vi "limit switch.vi"(9 "lower limit":bool, 10 "upper limit":bool, 11 "motor input":dbl) -> (3 "motor output":dbl)   [LabVIEW 2014]
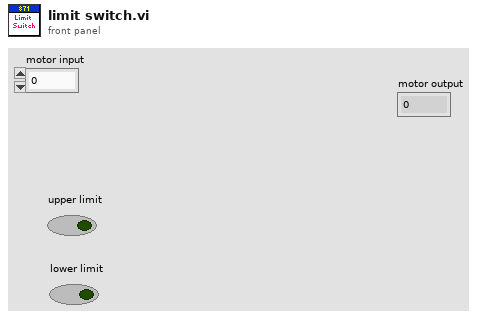
[diagram p1: front panel]
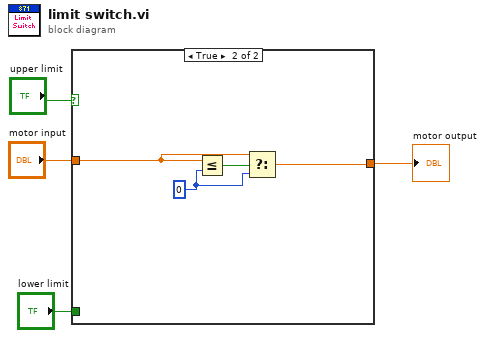
[diagram p0: block diagram]
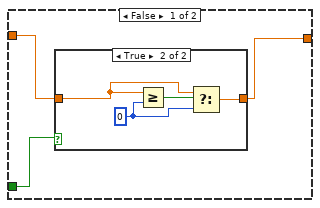
[diagram p2: hidden frame]
diagram:
  n1 = case shown="True" "upper limit" {
    tunnel: "motor input" -> [w6 w14]
    tunnel: [w5 w13] -> w4
    tunnel: "lower limit" -> [w7 _]
    frame False {
      n2 = case shown="True" w7 {
        tunnel: w6 -> [w8 w10]
        tunnel: [w8 w9] -> w5
        frame False {
        }
        frame True {
          w11 = 0
          n3 = Greater Or Equal?(x=w10, y=w11) -> (x >= y?=w12:bool)
          n4 = Select(t=w10, s=w12, f=w11) -> (s? t:f=w9:dbl)
        }
      }
    }
    frame True {
      w15 = 0
      n5 = Less Or Equal?(x=w14, y=w15) -> (x <= y?=w16:bool)
      n6 = Select(t=w14, s=w16, f=w15) -> (s? t:f=w13:dbl)
    }
  }
  "motor output" <- w4
